vi "KE622x -- Set RS-232 Params.vi"(0 "Resource In":refnum<visa-resource-name>, 1 "Check For SCPI Errors? (T)":bool=TRUE, 11 "error in (no error)":errorcluster, 12 "Term Char (0xA)":u8=10 format="%02x") -> (4 "Resource Out (dupl)":refnum<visa-resource-name>, 15 "error out":errorcluster)   [LabVIEW 2009, in "Keithley 622x.lvlib"]
uses:
  <instrlib>/Keithley 622x LV 2009/Keithley 622x.lvlib
  <instrlib>/Keithley 622x LV 2009/Utility/Typedefs/KE622x -- Serial Port Settings.ctl
panel:
  out "RS-232 Settings":T1={"Read Term Char"=enum."CR", "Baud Rate"=enum."19200", "Flow Control\n(XON / XOFF)"=enum."Off"}
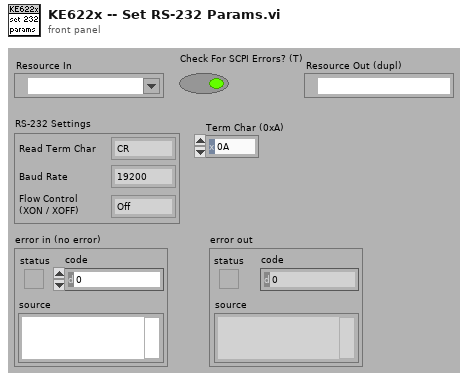
[diagram p1: front panel]
types:
  T1 = typedef "Keithley 622x.lvlib/KE622x -- Serial Port Settings.ctl" = cluster{"Read Term Char":enum16{"CR", "LF", "CR + LF", "LF + CR"}, "Baud Rate":enum16{"300", "600", "1200", "2400", "4800", "9600", "19200", "38400", "57600", "115200"}, "Flow Control\n(XON / XOFF)":enum16{"Off", "On"}}
  T2 = enum16{"300", "600", "1200", "2400", "4800", "9600", "19200", "38400", "57600", "115200"}
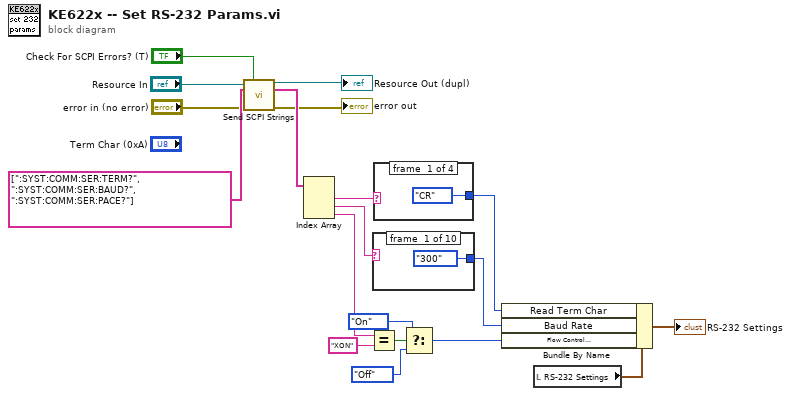
[diagram p0: block diagram]
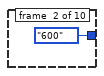
[diagram p2: hidden frame]
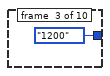
[diagram p3: hidden frame]
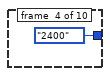
[diagram p4: hidden frame]
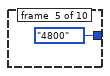
[diagram p5: hidden frame]
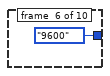
[diagram p6: hidden frame]
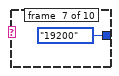
[diagram p7: hidden frame]
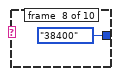
[diagram p8: hidden frame]
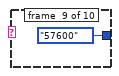
[diagram p9: hidden frame]
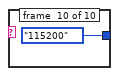
[diagram p10: hidden frame]
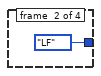
[diagram p11: hidden frame]
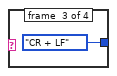
[diagram p12: hidden frame]
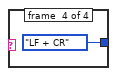
[diagram p13: hidden frame]
diagram:
  n1 = call <instrlib>:"Send SCPI Strings.vi"("Resource In"="Resource In", "Check For SCPI Errors? (T)"="Check For SCPI Errors? (T)", "SCPI Strings (no term char)"=string[] [":SYST:COMM:SER:TERM?", ":SYST:COMM:SER:BAUD?", ":SYST:COMM:SER:PACE?"], "error in (no error)"="error in (no error)") -> ("Resource Out (dupl)"=→"Resource Out (dupl)":refnum<visa-resource-name>, "Query Responses"=w15:string[], "error out"=→"error out":errorcluster)  [unwired: 8 in, 1 out]
  n2 = Index Array(array=w15) -> (element #1=w14:string, element #2=w12:string, element #3=w11:string)  [unwired: 3 in]
  n3 = Equal?(x=w11, y="XON") -> (x = y?=w8:bool)
  n4 = case shown="\"115200\"" w12 {
    tunnel: [T2."300" ("Baud Rate") T2."600" ("Baud Rate") T2."1200" ("Baud Rate") T2."2400" ("Baud Rate") T2."4800" ("Baud Rate") T2."9600" ("Baud Rate") T2."19200" ("Baud Rate") T2."38400" ("Baud Rate") T2."57600" ("Baud Rate") T2."115200" ("Baud Rate")] -> w1
    frame #0 {
    }
    frame #1 {
    }
    frame #2 {
    }
    frame #3 {
    }
    frame #4 {
    }
    frame #5 {
    }
    frame #6 {
    }
    frame #7 {
    }
    frame #8 {
    }
    frame #9 {
    }
  }
  n5 = case shown="\"LFCR\"" w14 {
    tunnel: [enum16{"CR", "LF", "CR + LF", "LF + CR"}."CR" ("Term Char") enum16{"CR", "LF", "CR + LF", "LF + CR"}."LF" ("Term Char") enum16{"CR", "LF", "CR + LF", "LF + CR"}."CR + LF" ("Term Char") enum16{"CR", "LF", "CR + LF", "LF + CR"}."LF + CR" ("Term Char")] -> w9
    frame #0 {
    }
    frame #1 {
    }
    frame #2 {
    }
    frame #3 {
    }
  }
  n6 = Select(t=enum16{"Off", "On"}."On", s=w8, f=enum16{"Off", "On"}."Off" ("Flow Control\n(XON / XOFF)")) -> (s? t:f=w5:enum16{"Off", "On"})
  n7 = local read "RS-232 Settings"() -> (w13:T1)
  n8 = Bundle By Name(cluster=w13, "Read Term Char"=w9, "Baud Rate"=w1, "Flow Control\n(XON / XOFF)"=w5) -> (→"RS-232 Settings":T1)
